vi "CheckResume.vi"(0 "error in":errorcluster) -> (1 "Resumed":bool, 3 "error out":errorcluster)   [LabVIEW 2020]
uses:
  Globals and TypeDefs/gGeneral.vi
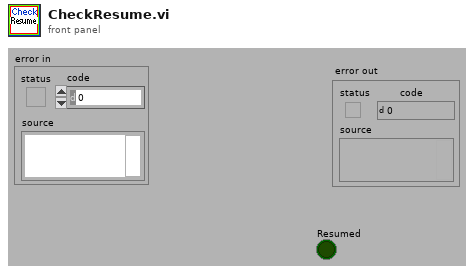
[diagram p1: front panel]
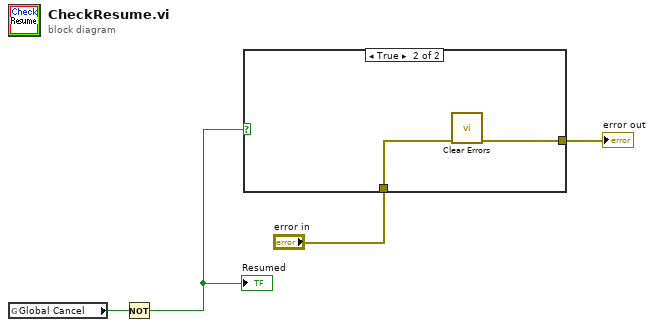
[diagram p0: block diagram]
diagram:
  n1 = global read "gGeneral.vi" "Global Cancel"() -> (w2:bool)
  n2 = Not(x=w2) -> (.not. x?=w1:bool)
  "Resumed" <- w1
  n3 = case shown="True" w1 {
    tunnel: [w5 w6] -> w4
    tunnel: "error in" -> [w5 w7]
    frame False {
    }
    frame True {
      n4 = call <vilib>:"Clear Errors.vi"("error in (no error)"=w7) -> ("error out"=w6:errorcluster)  [unwired: 5 in, 1 out]
    }
  }
  "error out" <- w4
